vi "ComconnInital.vi"(2 "error in":errorcluster caption="错误输入（无错误）", 3 "COMIn":refnum<visa-resource-name>) -> (0 "error out":errorcluster caption="错误输出", 1 "COMOut":refnum<visa-resource-name>)   [LabVIEW 2013]
uses:
  <vilib>/Instr/_visa.llb/VISA Flush IO Buffer Mask.ctl
  <vilib>/Instr/_visa.llb/VISA Configure Serial Port (Instr).vi
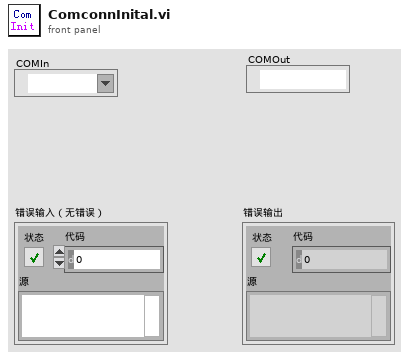
[diagram p1: front panel]
types:
  T1 = typedef "VISA Flush IO Buffer Mask.ctl" = u16
  T2 = cluster{"波特率":u32, "数据比特":u16, "奇偶":enum16{"None", "Odd", "Even", "Mark", "Space"}, "停止位":u16, "流控制":u16}
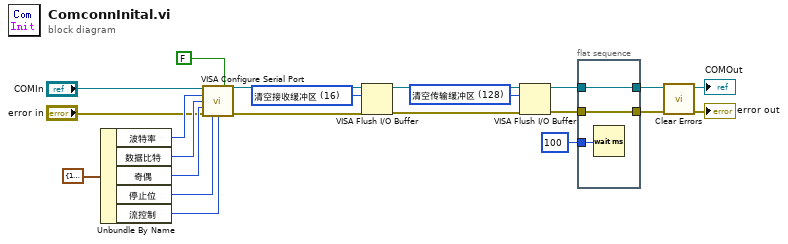
[diagram p0: block diagram]
diagram:
  w9 = T1 128 items=["清空接收缓冲区"=16, "向设备写入传输缓冲区"=32, "清空接收缓冲区（无I/O）"=64, "清空传输缓冲区"=128] ("Mask")
  w11 = T1 16 items=["清空接收缓冲区"=16, "向设备写入传输缓冲区"=32, "清空接收缓冲区（无I/O）"=64, "清空传输缓冲区"=128] ("Mask")
  n1 = Unbundle By Name(T2 {"波特率"=115200, "数据比特"=8, "奇偶"=enum."None", "停止位"=10, "流控制"=0} ("串口设置")) -> ("波特率"=w19:u32, "数据比特"=w18:u16, "奇偶"=w17:enum16{"None", "Odd", "Even", "Mark", "Space"}, "停止位"=w16:u16, "流控制"=w15:u16)
  n2 = call-poly "VISA Configure Serial Port"("VISA resource name"="COMIn", "Enable Termination\nChar (T)"=FALSE, "baud rate (9600)"=w19, "data bits (8)"=w18, "parity (0:none)"=w17, "error in (no error)"="error in", "stop bits (10: 1 bit)"=w16, "flow control (0:none)"=w15) -> ("VISA resource name out"=w13:refnum<visa-resource-name>, "error out"=w12:errorcluster)  [unwired: 6 in]
  n3 = VISA Flush I/O Buffer(VISA resource name=w13, mask (16)=w11, error in (no error)=w12) -> (VISA resource name out=w8:refnum<visa-resource-name>, error out=w7:errorcluster)
  n4 = VISA Flush I/O Buffer(VISA resource name=w8, mask (16)=w9, error in (no error)=w7) -> (VISA resource name out=w5:refnum<visa-resource-name>, error out=w2:errorcluster)
  n5 = flat-sequence {
    tunnel: [w24] -> w6
    tunnel: w5 -> [w24]
    tunnel: 100 -> [w23]
    tunnel: [w22] -> w3
    tunnel: w2 -> [w22]
    frame #0 {
      n6 = Wait (ms)(milliseconds to wait=w23) -> ()  [unwired: 1 out]
    }
  }
  n7 = call <vilib>:"Clear Errors.vi"("error in (no error)"=w3) -> ("error out"=→"error out":errorcluster)  [unwired: 6 in]
  "COMOut" <- w6
